vi "clean_raw_data_.vi"(8 "error in (no error)":errorcluster, 9 "data raw":cluster{"I":i32[][], "II":i32[][]}, 10 "N of scans":i32, 11 "VIS-NIR_STRESING_NEW in":refnum<class "VIS-NIR_STRESING_NEW.lvclass">) -> (0 "error out":errorcluster, 1 "I 2":i32[][](array[numeric]), 2 "I":i32[][](array[numeric]), 3 "VIS-NIR_STRESING_NEW out":refnum<class "VIS-NIR_STRESING_NEW.lvclass">)   [LabVIEW 2020, in "VIS-NIR_STRESING_NEW.lvclass"]
uses:
  VIS-NIR_STRESING_NEW.lvclass
panel:
  in  "exchange I and II":bool
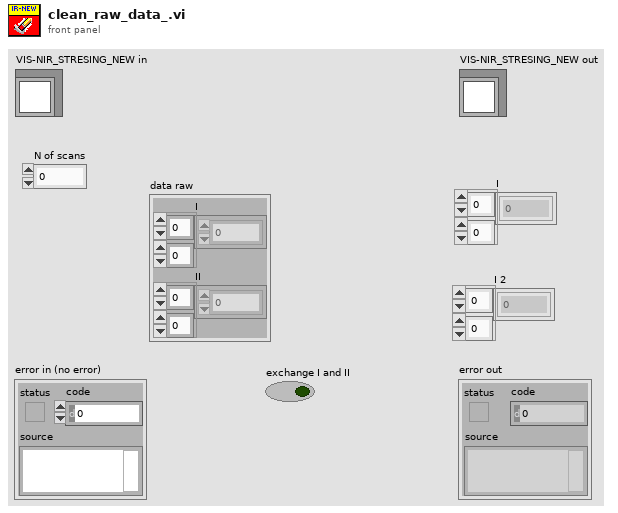
[diagram p1: front panel]
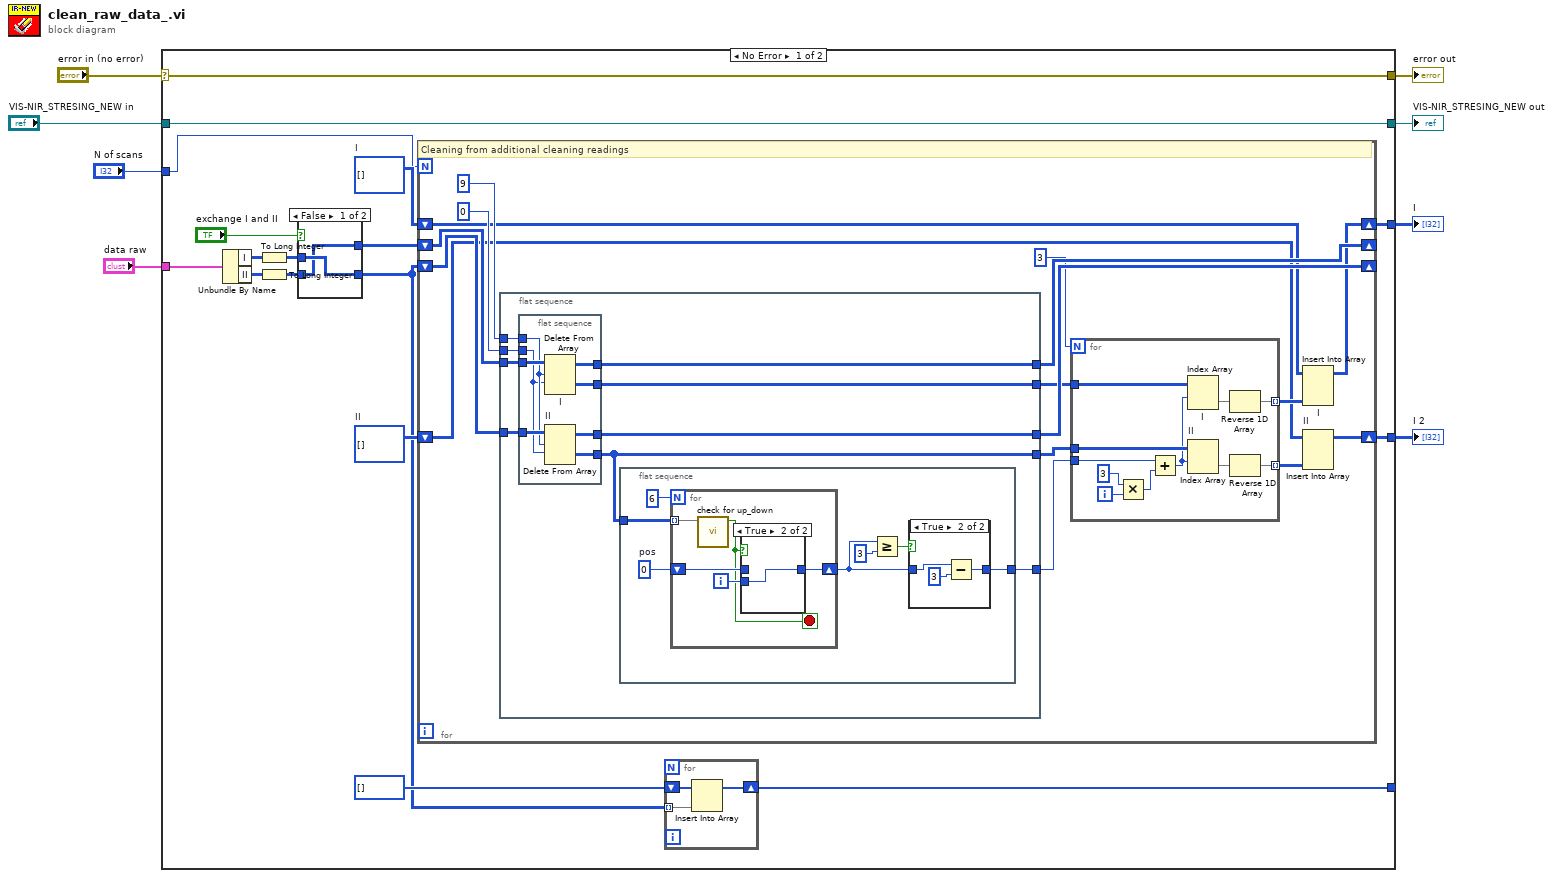
[diagram p0: block diagram]
diagram:
  n1 = case shown="No Error" "error in (no error)" {
    selector: "error in (no error)" -> [w16 w96]
    tunnel: [w16 w96] -> w4
    tunnel: [w25 w95] -> w6
    tunnel: "VIS-NIR_STRESING_NEW in" -> [w25 w95]
    tunnel: [w15 _] -> w3
    tunnel: [w14 _] -> w2
    tunnel: [w13 _] -> _
    tunnel: "N of scans" -> [w12 _]
    tunnel: "data raw" -> [w11 _]
    frame No Error {
      w24 = i32[][] []  # II
      w23 = i32[][] []  # I
      n2 = Unbundle By Name(w11) -> ("I"=w10:i32[][], "II"=w9:i32[][])
      n3 = To Long Integer(number=w10) -> (32bit integer=w21:i32[][])
      n4 = To Long Integer(number=w9) -> (32bit integer=w22:i32[][])
      n5 = case shown="False" "exchange I and II" {
        tunnel: [w88 w91] -> w18
        tunnel: w21 -> [w89 w91]
        tunnel: w22 -> [w88 w90]
        tunnel: [w89 w90] -> w19
        frame False {
        }
        frame True {
        }
      }
      n6 = for {
        N: w12 -> [_]
        shift-right: [w40] -> _
        shift-left: w18 -> [w41]
        shift-right: [w38] -> _
        shift-left: w19 -> [w39]
        shift-right: [w29] -> w15
        shift-left: w23 -> [w30]
        shift-right: [w26] -> w14
        shift-left: w24 -> [w27]
        # "Cleaning from additional cleaning readings"
        n7 = flat-sequence {
          tunnel: w41 -> [w50]
          tunnel: [w49] -> w40
          tunnel: w39 -> [w48]
          tunnel: [w47] -> w38
          tunnel: 9 ("length") -> [w46]
          tunnel: 0 ("index (row)") -> [w45]
          tunnel: [w44] -> w35
          tunnel: [w43] -> w34
          tunnel: [w42] -> w33
          frame #0 {
            n8 = flat-sequence {
              tunnel: w50 -> [w76]
              tunnel: [w75] -> w49
              tunnel: w48 -> [w74]
              tunnel: [w73] -> w47
              tunnel: w46 -> [w72]
              tunnel: w45 -> [w71]
              tunnel: [w70] -> w44
              tunnel: [w69] -> w43
              frame #0 {
                n9 = Delete From Array "I"(array=w76, length=w72, index (row)=w71) -> (deleted portion=w70:i32[][], array with subset deleted=w75:i32[][])  [unwired: 1 in]
                n10 = Delete From Array "II"(array=w74, length=w72, index (row)=w71) -> (deleted portion=w69:i32[][], array with subset deleted=w73:i32[][])  [unwired: 1 in]
              }
            }
            n11 = flat-sequence {
              tunnel: w43 -> [w52]
              tunnel: [w51] -> w42
              frame #0 {
                w56 = 0  # pos
                n12 = for {
                  N: 6 -> [_]
                  tunnel: w52 -> [w63] mode=indexing
                  shift-right: [w64] -> w54
                  shift-left: w56 -> [w66]
                  i -> [w65]
                  stop <- w62 stop-if-true
                  n13 = call "check for up_down.vi"("Array"=w63) -> ("Yes/No"=w62:bool)  [unwired: 10 in]
                  n14 = case shown="True" w62 {
                    tunnel: [w67 w68] -> w64
                    tunnel: w66 -> [w67 _]
                    tunnel: w65 -> [_ w68]
                    frame False {
                    }
                    frame True {
                    }
                  }
                }
                n15 = Greater Or Equal?(x=w54, y=3) -> (x >= y?=w53:bool)
                n16 = case shown="True" w53 {
                  tunnel: [w58 w59] -> w51
                  tunnel: w54 -> [w58 w61]
                  frame False {
                  }
                  frame True {
                    n17 = Subtract(x=w61, y=3) -> (x-y=w59:i32)
                  }
                }
              }
            }
          }
        }
        n18 = for {
          N: 3 -> [_]
          tunnel: w35 -> [w87]
          tunnel: w34 -> [w86]
          tunnel: w33 -> [w82]
          tunnel: [w77] -> w31 mode=indexing
          tunnel: [w79] -> w28 mode=indexing
          i -> [w85]
          n19 = Multiply(x=3, y=w85) -> (x*y=w83:i32)
          n20 = Add(x=w82, y=w83) -> (x+y=w81:i32)
          n21 = Index Array "I"(array=w87, index (row)=w81) -> (element=w78:i32[])  [unwired: 1 in]
          n22 = Index Array "II"(array=w86, index (row)=w81) -> (element=w80:i32[])  [unwired: 1 in]
          n23 = Reverse 1D Array(array=w78) -> (reversed array=w77:i32[])
          n24 = Reverse 1D Array(array=w80) -> (reversed array=w79:i32[])
        }
        n25 = Insert Into Array "I"(array=w30, new element=w31) -> (w29:i32[][])  [unwired: 2 in]
        n26 = Insert Into Array "II"(array=w27, new element=w28) -> (w26:i32[][])  [unwired: 2 in]
      }
      n27 = for {
        tunnel: w19 -> [w93] mode=indexing
        shift-right: [w92] -> w13
        shift-left: i32[] [] ("II RAW") -> [w94]
        n28 = Insert Into Array(array=w94, new element=w93) -> (w92:i32[])  [unwired: 1 in]
      }
    }
    frame Error {
    }
  }
  "error out" <- w4
  "VIS-NIR_STRESING_NEW out" <- w6
  "I" <- w3
  "I 2" <- w2
